vi "Read.vi"(8 "error in (no error)":errorcluster, 11 "Modbus PLC in":refnum<class "Modbus PLC.lvclass">) -> (0 "error out":errorcluster, 2 "Read Data":variant, 3 "Modbus PLC out":refnum<class "Modbus PLC.lvclass">)   [LabVIEW 2023, in "Modbus PLC.lvlib" / "Modbus PLC.lvclass"]
uses:
  Modbus PLC.lvclass
  Data.ctl
  Modbus PLC.lvclass/Modbus PLC.ctl
  <vilib>/NI/Modbus Library/API/Master/Modbus Master.lvclass
panel:
  out "IND":T1 {"Rotate_IND" items=["стоп", "Качалка Режим Авто", "Качалка Режим Ручной"]; "Termex_IND" items=["Термостат старт"=1, "Термостат стоп"=0]; "Mix_IND" items=["Мешалка движение вперёд"=1, "Мешалка движение назад"=2, "Мешалка стоп"=0]}
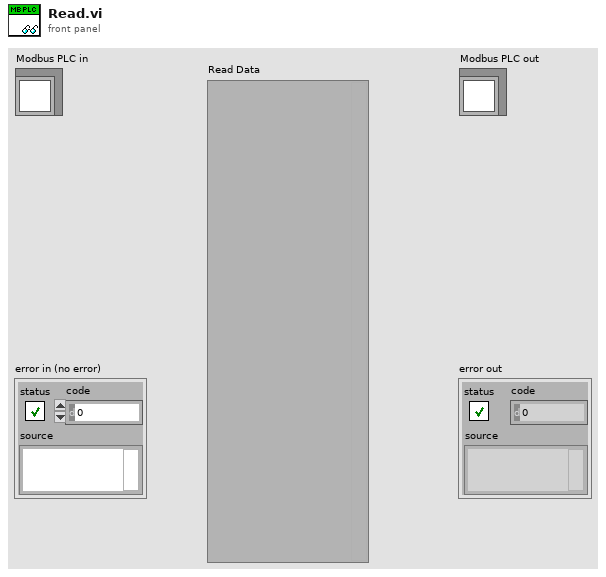
[diagram p1: front panel]
types:
  T1 = typedef "Modbus PLC.lvlib/Modbus PLC.lvclass/Data.ctl" = cluster{"Rotate_IND":u16, "Termex_IND":u16, "Mix_IND":u16, "Rotate_PV_Angle_Init":u16, "Rotate_PV_Angle_End":u16, "Rotate_PV_Timeout":u16, "Rotate_PV_Speed":u16, "Rotate_PV_Time":u16, "Rotate_PV_Angle":u16, "Termex_SP":sgl, "MIX_PV":u16, "Termex_PV_In":sgl, "Termex_KP":sgl, "P_PV":sgl, "Termex_PV_Out":sgl, "Termex_TN":sgl, "MM_PV":sgl}
  T2 = typedef "Modbus PLC.lvlib/Modbus PLC.lvclass/Output Map.ctl" = map{string, cluster{"Address":i32, "Data Type":enum16{"Int", "Float"}, "Reg Type":enum16{"Holding", "Input", "Coil"}}}
  T3 = cluster{"Address":i32, "Data Type":enum16{"Int", "Float"}, "Reg Type":enum16{"Holding", "Input", "Coil"}}
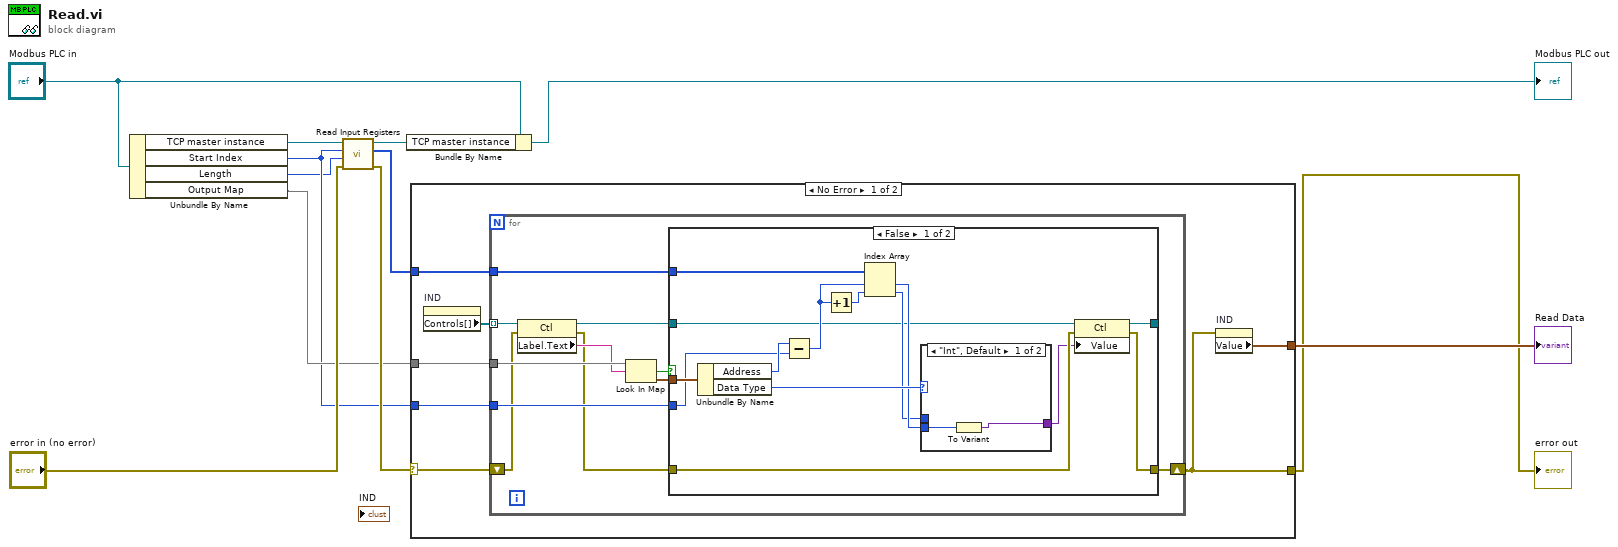
[diagram p0: block diagram]
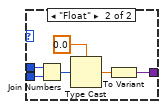
[diagram p2: hidden frame]
diagram:
  n1 = Unbundle By Name("Modbus PLC in") -> ("TCP master instance"=w12:refnum<class "Modbus Master.lvclass">, "Start Index"=w5:u16, "Length"=w3:u16, "Output Map"=w6:T2)
  n2 = call-dynamic "Read Input Registers.vi"("error in"="error in (no error)", "number of inputs"=w3, "starting address"=w5, "Modbus master in"=w12) -> ("error out"=w10:errorcluster, "register values"=w7:u16[], "Modbus master out"=w8:refnum<class "Modbus Master.lvclass">)  [unwired: 5 in]
  n3 = Bundle By Name(cluster="Modbus PLC in", "TCP master instance"=w8) -> (→"Modbus PLC out":refnum<class "Modbus PLC.lvclass">)
  n4 = case shown="No Error" w10 {
    selector: w10 -> [w15 w55]
    tunnel: w7 -> [w18 _]
    tunnel: w6 -> [w17 _]
    tunnel: w5 -> [w16 _]
    tunnel: [w13 w55] -> w1
    tunnel: [w14 _] -> w4
    frame No Error {
      n5 = property on="IND" class="Clust (strict)"() -> ("Controls[]"=w19:refnum<vi>[])  [unwired: 2 in, 2 out]
      n6 = for {
        tunnel: w19 -> [w30] mode=indexing
        tunnel: w18 -> [w25]
        tunnel: w17 -> [w29]
        tunnel: w16 -> [w26]
        shift-right: [w22] -> w13
        shift-left: w15 -> [w23]
        n7 = property class="Ctl"(reference=w30, error in=w23) -> (reference out=w24:refnum<vi>, error out=w21:errorcluster, "Label.Text"=w28:string)
        n8 = Look In Map(map=w29, key=w28) -> (key not found?=w20:bool, value=w27:T3)  [unwired: 1 in]
        n9 = case shown="False" w20 {
          tunnel: w27 -> [w44 _]
          tunnel: w26 -> [w42 _]
          tunnel: w25 -> [w41 _]
          tunnel: w24 -> [w35 w53]
          tunnel: [w33 w54] -> w22
          tunnel: w21 -> [w34 w54]
          tunnel: [w32 w53] -> _
          frame False {
            n10 = Unbundle By Name(w44) -> ("Address"=w43:i32, "Data Type"=w38:enum16{"Int", "Float"})
            n11 = Subtract(x=w43, y=w42) -> (x-y=w39:i32)
            n12 = Increment(x=w39) -> (x+1=w40:i32)
            n13 = Index Array(array=w41, index #1=w39, index #2=w40) -> (element #1=w37:u16, element #2=w36:u16)
            n14 = case shown="\"Int\", Default" w38 {
              tunnel: w37 -> [w46 w52]
              tunnel: w36 -> [_ w51]
              tunnel: [w45 w47] -> w31
              frame "Int", Default {
                n15 = To Variant(anything=w46) -> (Variant=w45:variant)
              }
              frame "Float" {
                n16 = Join Numbers(hi=w51, lo=w52) -> ((hi.lo)=w50:u32)
                n17 = Type Cast(type=sgl 0.0, x=w50) -> (*(type *) &x=w48:sgl)
                n18 = To Variant(anything=w48) -> (Variant=w47:variant)
              }
            }
            n19 = property class="Ctl"(reference=w35, error in=w34, "Value"=w31) -> (reference out=w32:refnum<vi>, error out=w33:errorcluster)
          }
          frame True {
          }
        }
      }
      n20 = property on="IND" class="Clust (strict)"(error in=w13) -> ("Value"=w14:T1)  [unwired: 1 in, 2 out]
    }
    frame Error {
    }
  }
  "error out" <- w1
  "Read Data" <- w4
